vi "Load_Table.vi"(8 "Error In":errorcluster) -> (0 "Error Out":errorcluster, 3 "MAC & Name Out":string[][](array[string]))   [LabVIEW 2017]
uses:
  <vilib>/Utility/file.llb/Read Delimited Spreadsheet (string).vi
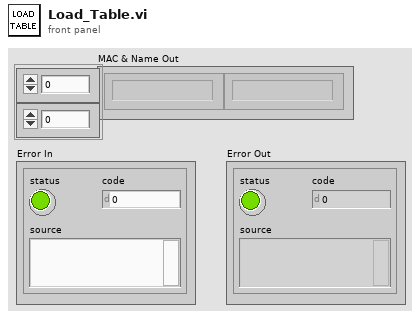
[diagram p1: front panel]
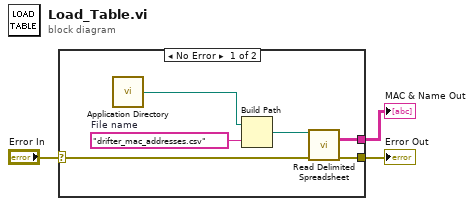
[diagram p0: block diagram]
diagram:
  n1 = case shown="No Error" "Error In" {
    selector: "Error In" -> [w5 w10]
    tunnel: [w6 _] -> w1
    tunnel: [w4 w10] -> w3
    frame No Error {
      w9 = "drifter_mac_addresses.csv"  # File name
      n2 = call <vilib>:"Application Directory.vi"() -> ("Application Directory"=w8:path)
      n3 = Build Path(base path=w8, name or relative path=w9) -> (appended path=w7:path)
      n4 = call-poly <vilib>:"Read Delimited Spreadsheet.vi"("file path (dialog if empty)"=w7, "error in (no error)"=w5) -> ("all rows"=w6:string[][], "error out"=w4:errorcluster)  [unwired: 8 in, 4 out]
    }
    frame Error {
    }
  }
  "Error Out" <- w3
  "MAC & Name Out" <- w1
